vi "Write4WirexVDTParameters.vi"(8 "error in (no error)":errorcluster, 9 "UserValues":dbl[](array[numeric]), 10 "4 Wire xVDT Parameters  in":T1[](array[typedef]), 11 "FPGA Session":u32) -> (0 "error out":errorcluster, 2 "4 Wire xVDT Parameters out":T1[](array[typedef]), 3 "FPGA Session Out":u32)   [LabVIEW 2011, in "Sensor Simulation Custom Device.lvlib"]
uses:
  Sensor Simulation Custom Device.lvlib
  TypeDefs/4 Wire xVDT Parameters.ctl
  <userlib>/_FPGA Interface Advanced Tools/FPGA Interface Wrapper/NiFPGA Write - I32.vi
  <vilib>/Utility/error.llb/Error Cluster From Error Code.vi
  <userlib>/_FPGA Interface Advanced Tools/FPGA Interface Wrapper/FPGA Interface Wrapper.lvlib
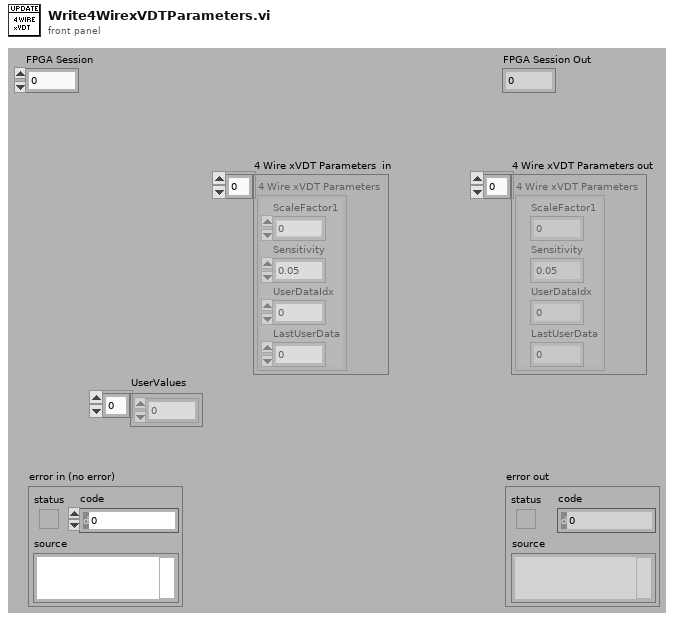
[diagram p1: front panel]
types:
  T1 = typedef "Sensor Simulation Custom Device.lvlib/4 Wire xVDT Parameters.ctl" = cluster{"ScaleFactor1":u32, "Sensitivity":dbl, "UserDataIdx":i32, "LastUserData":dbl}
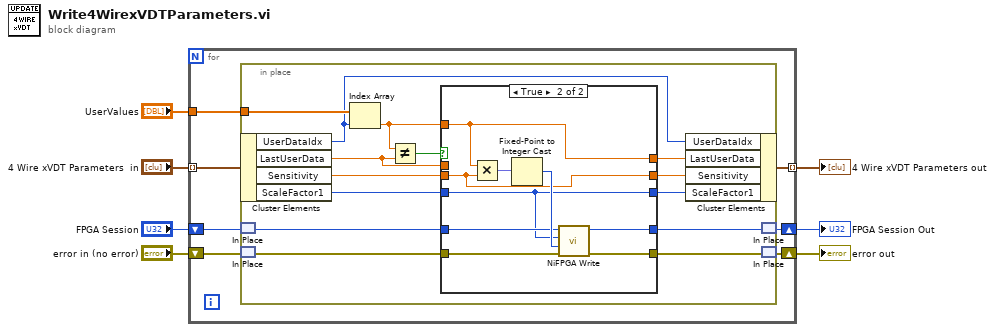
[diagram p0: block diagram]
diagram:
  n1 = for {
    shift-right: [w10] -> w6
    shift-left: "error in (no error)" -> [w13]
    shift-right: [w11] -> w5
    shift-left: "FPGA Session" -> [w12]
    tunnel: "4 Wire xVDT Parameters  in" -> [w9] mode=indexing
    tunnel: "UserValues" -> [w14]
    tunnel: [w8] -> w1 mode=indexing
    n2 = in-place {
      in-place-border: w14 -> [w28]
      n3 = in-place-cluster #1(w9) -> ("UserDataIdx"=w18:i32, "LastUserData"=w15:dbl, "Sensitivity"=w23:dbl, "ScaleFactor1"=w22:u32)
      n4 = in-place-match #2(w12) -> (w26:u32)
      n5 = in-place-match #3(w13) -> (w27:errorcluster)
      n6 = Index Array(array=w28, index=w18) -> (element=w20:dbl)
      n7 = Not Equal?(x=w20, y=w15) -> (x != y?=w21:bool)
      n8 = case shown="True" w21 {
        tunnel: w27 -> [w30 w40]
        tunnel: w26 -> [w29 w39]
        tunnel: [w29 w38] -> w25
        tunnel: [w30 w37] -> w24
        tunnel: w23 -> [w32 w34]
        tunnel: w22 -> [w33 w35]
        tunnel: w20 -> [_ w36]
        tunnel: [w31 w36] -> w19
        tunnel: [w33 w35] -> w17
        tunnel: [w32 w34] -> w16
        tunnel: w15 -> [w31 _]
        frame False {
        }
        frame True {
          n9 = Multiply(x=w36, y=w34) -> (x*y=w42:fxp<+/-,19,5>)
          n10 = Fixed-Point to Integer Cast(1:w42) -> (0:w41:i32)
          n11 = call-poly <userlib>:"NiFPGA Write.vi"("error in (no error)"=w40, "Value"=w41, "Control"=w35, "Session"=w39) -> ("error out"=w37:errorcluster, "Session Out"=w38:u32)  [unwired: 6 in]
        }
      }
      n12 = in-place-cluster #1("UserDataIdx"=w18, "LastUserData"=w19, "Sensitivity"=w16, "ScaleFactor1"=w17) -> (w8:T1)
      n13 = in-place-match #2(w25) -> (w11:u32)
      n14 = in-place-match #3(w24) -> (w10:errorcluster)
    }
  }
  "error out" <- w6
  "FPGA Session Out" <- w5
  "4 Wire xVDT Parameters out" <- w1
